vi "ma_computeExpTimeConstant(samples).vi"(4 "dt":dbl format="%0.2f", 5 "averaging type":enum16{"Linear", "Exponential"}(ring), 6 "num Points":i32, 7 "reset":bool, 8 "error in (no error)":errorcluster, 9 "averaging time":dbl=-1.0 format="%0.2p", 10 "exp. time constant":dbl format="%0.2f", 11 "state info":T1 {"buffer" format="%0.2f"; "timestamp" format="%<%.4X>T"; "dt history" format="%0.2f"; "t0 history" format="%<%I:%M:%S%4u %p>T"; "exp TC (samples)" format="%0.2f"; "RMS history" format="%0.2f"; "DC history" format="%0.2f"}) -> (0 "error out":errorcluster, 3 "state info":T1 {"buffer" format="%0.2f"; "timestamp" format="%<%.4X>T"; "dt history" format="%0.2f"; "t0 history" format="%<%I:%M:%S%4u %p>T"; "exp TC (samples)" format="%0.2f"; "RMS history" format="%0.2f"; "DC history" format="%0.2f"})   [LabVIEW 2020, in "NI_MAPro.lvlib"]
uses:
  NI_MAPro.lvlib
  NI_MABase.lvlib
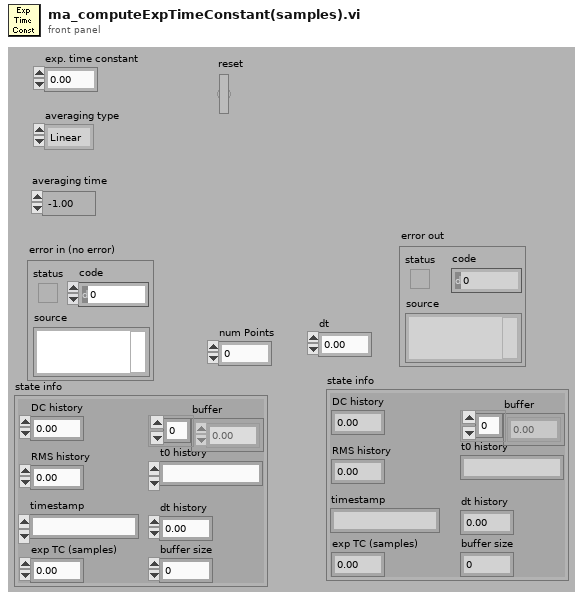
[diagram p1: front panel]
types:
  T1 = cluster{"DC history":dbl, "RMS history":dbl, "exp TC (samples)":dbl, "buffer size":i32, "t0 history":timestamp, "dt history":dbl, "timestamp":timestamp, "buffer":dbl[]}
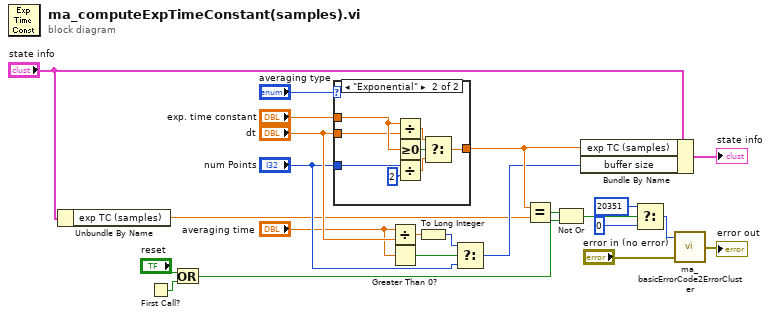
[diagram p0: block diagram]
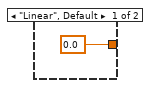
[diagram p2: hidden frame]
diagram:
  n1 = Unbundle By Name("state info") -> ("exp TC (samples)"=w6:dbl)
  n2 = First Call?() -> (First Call?: T/F=w19:bool)
  n3 = Or(x="reset", y=w19) -> (x .or. y?=w17:bool)
  n4 = case shown="\"Exponential\"" "averaging type" {
    tunnel: "exp. time constant" -> [_ w27]
    tunnel: "num Points" -> [_ w28]
    tunnel: [0.0 w26] -> w21
    tunnel: "dt" -> [_ w25]
    frame "Linear", Default {
    }
    frame "Exponential" {
      n5 = Divide(x=w27, y=w25) -> (x/y=w31:dbl)
      n6 = Greater Or Equal To 0?(x=w27) -> (x >= 0?=w32:bool)
      n7 = Divide(x=w28, y=2) -> (x/y=w30:dbl)
      n8 = Select(t=w31, s=w32, f=w30) -> (s? t:f=w26:dbl)
    }
  }
  n9 = Divide(x="averaging time", y="dt") -> (x/y=w3:dbl)
  n10 = Greater Than 0?(x="averaging time") -> (x > 0?=w2:bool)
  n11 = To Long Integer(number=w3) -> (32bit integer=w1:i32)
  n12 = Select(t=w1, s=w2, f="num Points") -> (s? t:f=w20:i32)
  n13 = Equal?(x=w21, y=w6) -> (x = y?=w10:bool)
  n14 = Not Or(1:w17, 2:w10) -> (0:w13:bool)
  n15 = Bundle By Name(cluster="state info", "exp TC (samples)"=w21, "buffer size"=w20) -> (→"state info":T1)
  n16 = Select(t=20351 ("code"), s=w13, f=0 ("code")) -> (s? t:f=w9:i32)
  n17 = call "ma_basicErrorCode2ErrorCluster.vi"("error in (no error)"="error in (no error)", "Error Code"=w9) -> ("error out"=→"error out":errorcluster)  [unwired: 1 in]
